vi "DoublePulse_Delay_Scan_Setup.vi"(7 "Rep. Rate (Hz)":dbl=10.0 min=0.0 max=34.0, 9 "ZeroDelayPos":dbl caption="Zero Delay \nPosition (mm)" format="%#.3f", 10 "Start Position":dbl[](array[numeric]) min=0.0 max=34.0, 11 "ESP300":refnum<queue>) -> (0 "Laser_Ctrl":bool, 1 "start/end points":cluster{dbl, dbl, dbl}[][](array[cluster]), 2 "Canceled":bool, 3 "SecondaryParams":variant[](array[variant]), 5 "ImageParameter":T1)   [LabVIEW 2013]
uses:
  ImagingMS/ImageConvPara.ctl
  <instrlib>/ESP300/Public/Data/ESP300_State.ctl
  <instrlib>/ESP300/ESP300.lvlib
panel:
  out "Delay Points":dbl[](array[numeric])
  in  "Step#2":i32=60 min=0
  in  "Delay Step 2":dbl=5.0
  in  "Step#1":i32=4 min=0
  in  "Delay Step (ps)":dbl=0.01 min=0.0 max=34.0
  in  "X StepWidth":dbl=0.05 min=0.0 max=34.0
  in  "LaserCtrl":bool
  out "Estimated Time (min)":dbl min=0.0 max=34.0
  in  "Average/pixel":i32=10 min=0 max=34
  in  "Cancel":bool
  in  "Run":bool
  out "XY Graph":cluster{dbl, dbl, "X StepWidth":dbl}[](graph)
  out "Y Size (mm)":dbl min=0.0 max=34.0
  out "X Size (mm)":dbl min=0.0 max=34.0
  out "Y Steps":i32=50 min=0 max=34
  in  "X Size":dbl=1.0 min=0.0 max=34.0
  in  "Y StepWidth":dbl=0.05 min=0.0 max=34.0
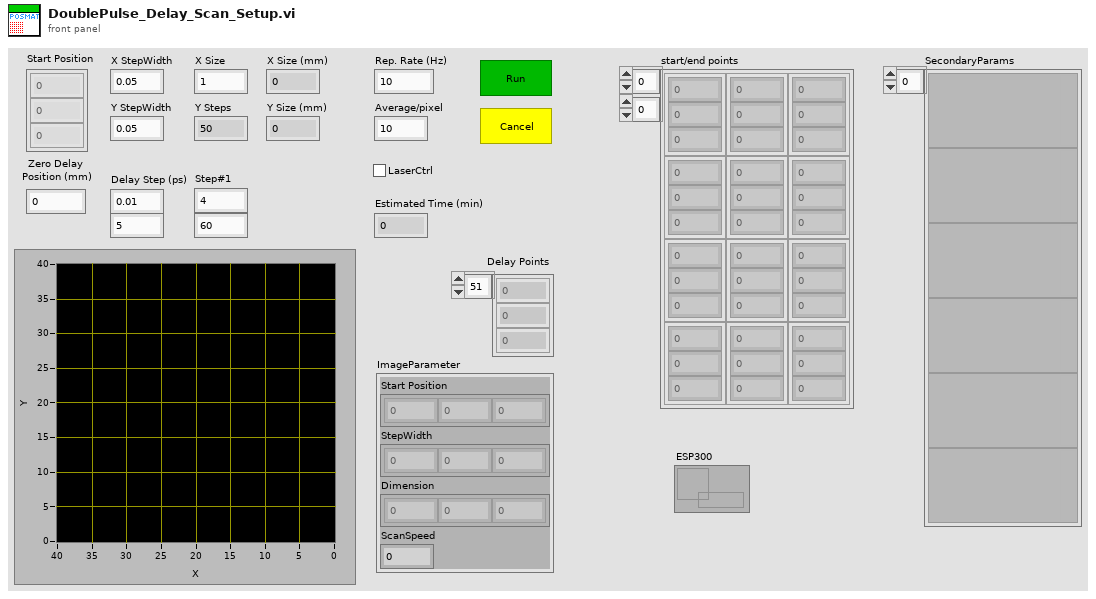
[diagram p1: front panel]
types:
  T1 = typedef "ImageConvPara.ctl" = cluster{"Start Position":dbl[], "StepWidth":dbl[], "Dimension":i32[], "ScanSpeed":dbl}
  T2 = cluster{"MotionStageRefs":refnum<queue>, "Axis#":i32, "Delay(ps)":dbl, "ZeroDelay_Offset":dbl}
  T3 = cluster{"MotionStageRefs":refnum<queue>, "Axis#":i32, "Delay(ps)":dbl, "ZeroDelay_Offset":dbl}[]
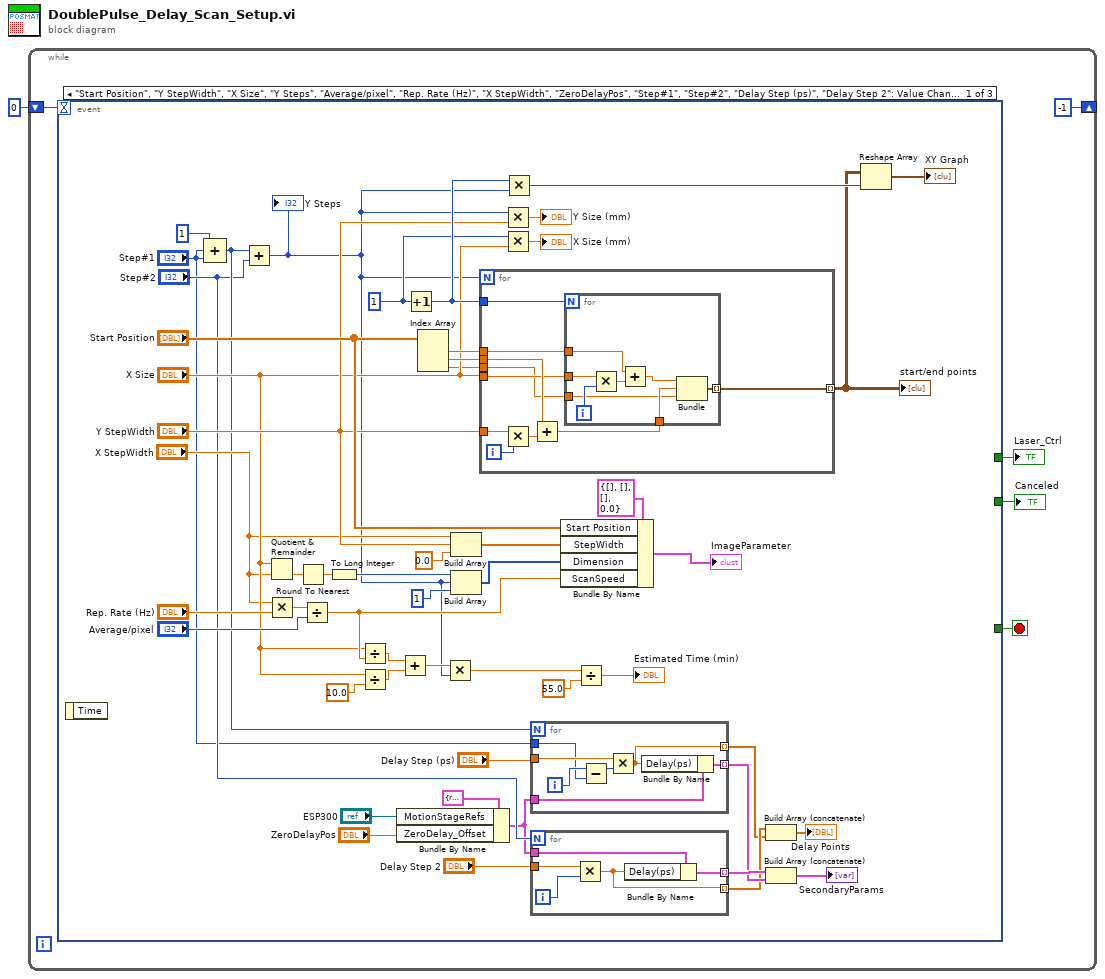
[diagram p0: block diagram]
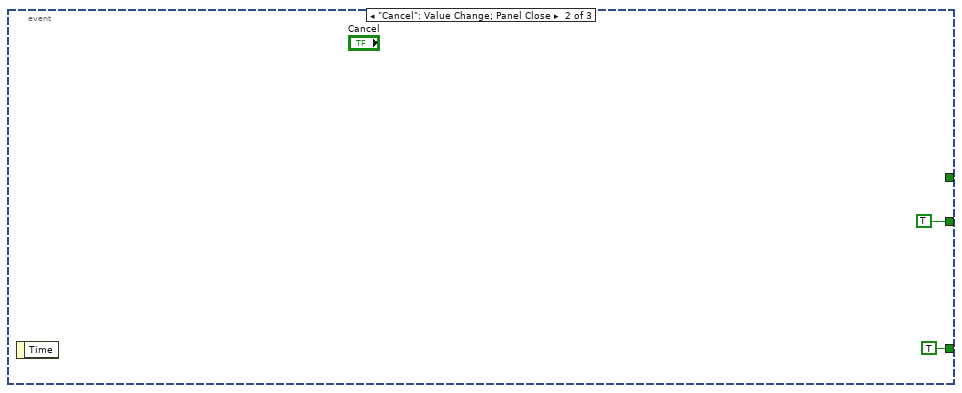
[diagram p2: hidden frame]
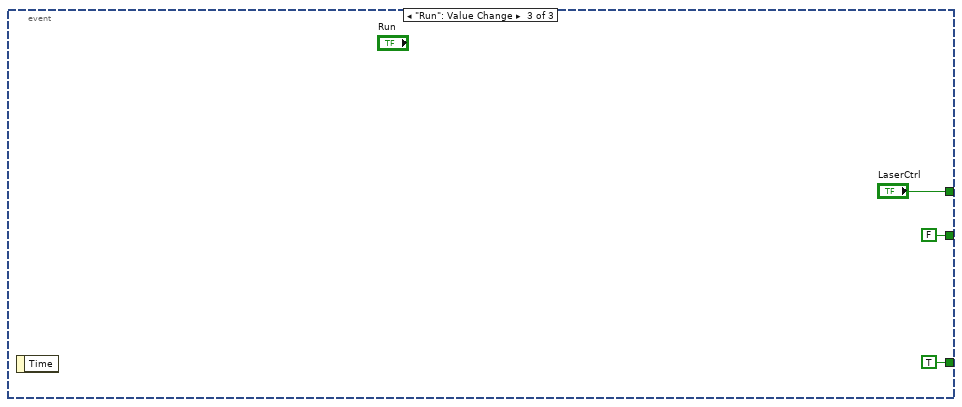
[diagram p3: hidden frame]
diagram:
  n1 = while {
    shift-right: [-1] -> _
    shift-left: 0 -> [w3]
    stop <- w6 stop-if-true
    n2 = event shown="[0] \"Start Position\", \"Y StepWidth\", \"X Size\", \"Y Steps\", \"Average/pixel\", \"Rep. Rate (Hz)\", \"X StepWidth\", \"ZeroDelayPos\", \"Step#1\", \"Step#2\", \"Delay Step (ps)\", \"Delay Step 2\": Value Change;  Timeout" {
      selector: _ -> [_ _ _]
      dyn-events: _ -> [_ _ _]
      timeout: w3 -> [_ _ _]
      tunnel: [_ TRUE TRUE] -> w6
      tunnel: [_ TRUE ("Canceled") FALSE ("Canceled")] -> w5
      tunnel: [_ _ "LaserCtrl"] -> w4
      event "Start Position", "Y StepWidth", "X Size", "Y Steps", "Average/pixel", "Rep. Rate (Hz)", "X StepWidth", "ZeroDelayPos", "Step#1", "Step#2", "Delay Step (ps)", "Delay Step 2": Value Change; Timeout {
        w51 = 1
        n3 = event-data() -> ()  [unwired: 1 in, 1 out]
        n4 = Compound Arithmetic op=ADD(1 ("value"), "Step#1", "Step#1") -> (w15:i32)
        n5 = Add(x=w15, y="Step#2") -> (x+y=w17:i32)
        "Y Steps" <- w17
        n6 = Quotient & Remainder(x="X Size", y="X StepWidth") -> (floor(x/y)=w43:dbl)  [unwired: 1 out]
        n7 = Multiply(x="X StepWidth", y="Rep. Rate (Hz)") -> (x*y=w42:dbl)
        n8 = Round To Nearest(number=w43) -> (nearest integer value=w27:dbl)
        n9 = Divide(x=w42, y="Average/pixel") -> (x/y=w38:dbl)
        n10 = To Long Integer(number=w27) -> (32bit integer=w28:i32)
        n11 = Divide(x="X Size", y=w38) -> (x/y=w36:dbl)
        n12 = Divide(x="X Size", y=10.0) -> (x/y=w35:dbl)
        n13 = Bundle By Name(cluster=T2 {"MotionStageRefs"=refnum, "Axis#"=0, "Delay(ps)"=0.0, "ZeroDelay_Offset"=0.0} ("Params."), "MotionStageRefs"="ESP300", "ZeroDelay_Offset"="ZeroDelayPos") -> (w13:T2)
        n14 = Add(x=w36, y=w35) -> (x+y=w34:dbl)
        n15 = Increment(x=w51) -> (x+1=w52:i32)
        n16 = Index Array(array="Start Position") -> (element #1=w57:dbl, element #2=w56:dbl, element #3=w29:dbl)  [unwired: 3 in]
        n17 = Multiply(x=w34, y=w17) -> (x*y=w33:dbl)
        n18 = Build Array("X StepWidth", "Y StepWidth", 0.0 ("element")) -> (w46:dbl[])
        n19 = Build Array(w28, w17, 1 ("element")) -> (w45:i32[])
        n20 = for {
          N: w17 -> [_]
          tunnel: w56 -> [w74]
          tunnel: "Y StepWidth" -> [w70]
          tunnel: "X Size" -> [w73]
          tunnel: w52 -> [w76]
          tunnel: [w75] -> w49 mode=indexing
          tunnel: w29 -> [w71]
          tunnel: w57 -> [w72]
          i -> [w79]
          n21 = Multiply(x=w70, y=w79) -> (x*y=w78:dbl)
          n22 = Add(x=w74, y=w78) -> (x+y=w77:dbl)
          n23 = for {
            N: w76 -> [_]
            tunnel: w73 -> [w85]
            tunnel: w72 -> [w80]
            tunnel: w77 -> [w83]
            tunnel: [w84] -> w75 mode=indexing
            tunnel: w71 -> [w81]
            i -> [w86]
            n24 = Multiply(x=w85, y=w86) -> (x*y=w87:dbl)
            n25 = Add(x=w80, y=w87) -> (x+y=w82:dbl)
            n26 = Bundle(w82, w83, "X StepWidth"=w81) -> (w84:cluster{dbl, dbl, "X StepWidth":dbl})  [unwired: 1 in]
          }
        }
        "start/end points" <- w49
        n27 = Multiply(x=w17, y="Y StepWidth") -> (x*y=→"Y Size (mm)":dbl)
        n28 = Multiply(x=w51, y="X Size") -> (x*y=→"X Size (mm)":dbl)
        n29 = Multiply(x=w52, y=w17) -> (x*y=w53:i32)
        n30 = for {
          N: w15 -> [_]
          tunnel: w13 -> [w64]
          tunnel: "Delay Step (ps)" -> [w62]
          tunnel: [w61] -> w10 mode=indexing
          tunnel: "Step#1" -> [w59]
          tunnel: [w58] -> w8 mode=indexing
          i -> [w63]
          n31 = Subtract(x=w63, y=w59) -> (x-y=w60:i32)
          n32 = Multiply(x=w62, y=w60) -> (x*y=w58:dbl)
          n33 = Bundle By Name(cluster=w64, "Delay(ps)"=w58) -> (w61:T2)
        }
        n34 = for {
          N: "Step#2" -> [_]
          tunnel: w13 -> [w69]
          tunnel: "Delay Step 2" -> [w68]
          tunnel: [w67] -> w20 mode=indexing
          tunnel: [w66] -> w9 mode=indexing
          i -> [w65]
          n35 = Multiply(x=w68, y=w65) -> (x*y=w66:dbl)
          n36 = Bundle By Name(cluster=w69, "Delay(ps)"=w66) -> (w67:T2)
        }
        n37 = Bundle By Name(cluster=T1 {"Start Position"=[], "StepWidth"=[], "Dimension"=[], "ScanSpeed"=0.0} ("ImageParameter"), "Start Position"="Start Position", "StepWidth"=w46, "Dimension"=w45, "ScanSpeed"=w38) -> (→"ImageParameter":T1)
        n38 = Divide(x=w33, y=55.0) -> (x/y=→"Estimated Time (min)":dbl)
        n39 = Build Array (concatenate)(w9, w8) -> (→"Delay Points":dbl[])
        n40 = Build Array (concatenate)(w20, w10) -> (→"SecondaryParams":T3)
        n41 = Reshape Array(w49, w53) -> (→"XY Graph":cluster{dbl, dbl, "X StepWidth":dbl}[])
      }
      event "Cancel": Value Change; Panel Close {
        n42 = event-data() -> ()  [unwired: 1 in, 1 out]
      }
      event "Run": Value Change {
        n43 = event-data() -> ()  [unwired: 1 in, 1 out]
      }
    }
    "Canceled" <- w5
    "Laser_Ctrl" <- w4
  }
